vi "Clear Mutation History of lvClass.vi"(8 "error in (no error)":errorcluster, 11 "Path":path=path "D:/OneDrive - NI/_WorkingOn/CSM/Communicable-State-Machine/src/user.lib/_NEVSTOP/Communicable State Machine(CSM)/_Support/Priority Queue/Priority Queue.lvclass") -> (0 "error out":errorcluster, 2 "Mutation History":T1 {"LabVIEW Version" format="%.0x"})   [LabVIEW 2017]
doc: "Clears the mutation history stored in the LabVIEW class at Path and returns the history records that were removed."
uses:
  <vilib>/Utility/EditLVLibs/LVClass/Mutation History.ctl
  <vilib>/Utility/EditLVLibs/LVClass/Mutation Record.ctl
  <vilib>/Utility/EditLVLibs/LibVersion.ctl
  <vilib>/Utility/EditLVLibs/Edit LVLibs.lvlib
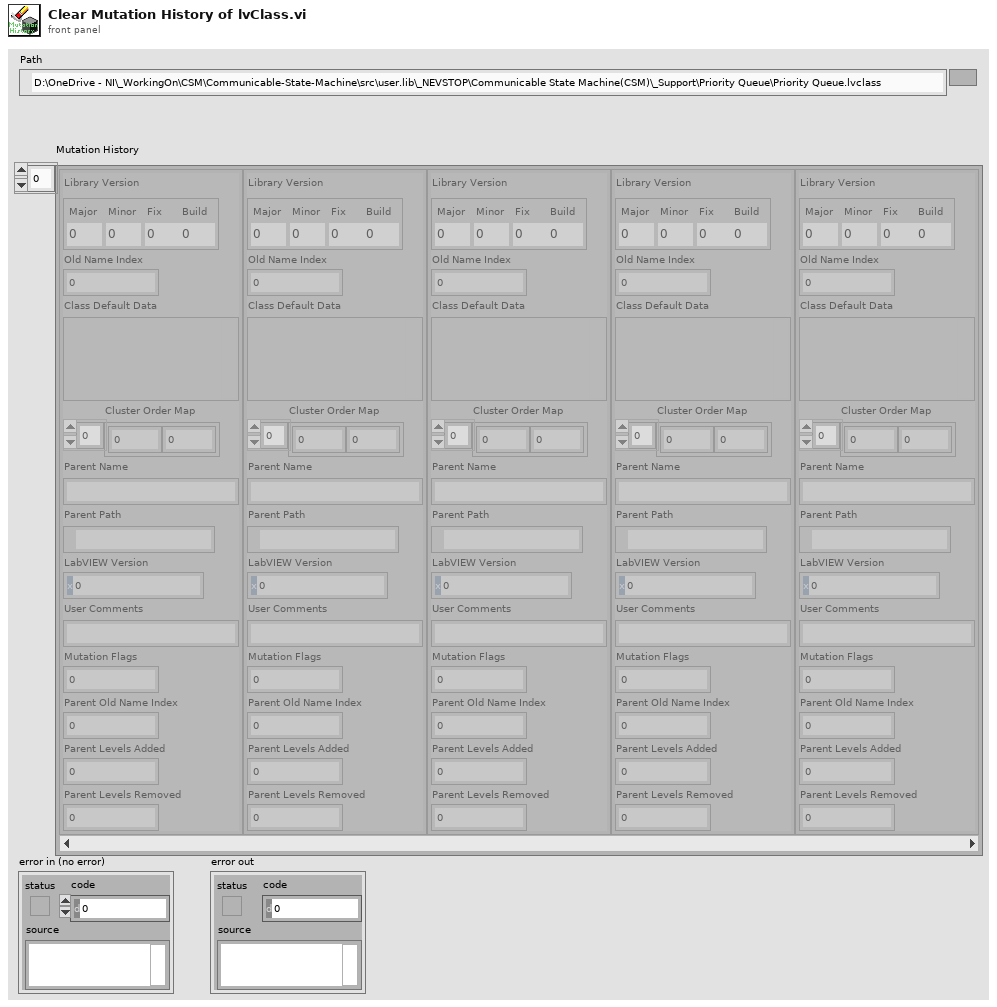
[diagram p1: front panel]
types:
  T1 = typedef "Edit LVLibs.lvlib/Mutation History.ctl" = T2[]
  T2 = typedef "Edit LVLibs.lvlib/Mutation Record.ctl" = cluster{"Library Version":T3, "Old Name Index":u8, "Class Default Data":variant, "Cluster Order Map":u32[], "Parent Name":string, "Parent Path":path, "LabVIEW Version":u32, "User Comments":string, "Mutation Flags":u8, "Parent Old Name Index":u8, "Parent Levels Added":u16, "Parent Levels Removed":u16}
  T3 = typedef "Edit LVLibs.lvlib/LibVersion.ctl" = cluster{"Major":u16, "Minor":u16, "Fix":u16, "Build":u16}
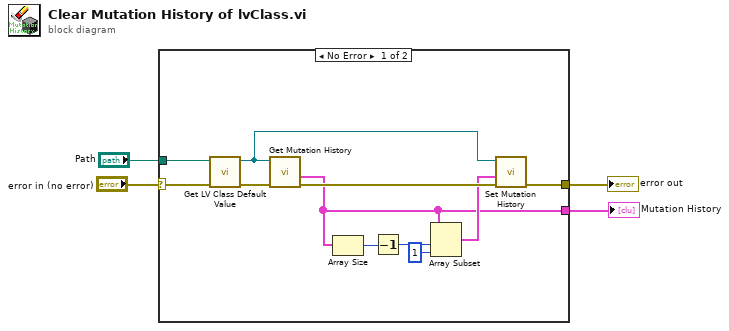
[diagram p0: block diagram]
diagram:
  n1 = case shown="No Error" "error in (no error)" {
    selector: "error in (no error)" -> [w6 w16]
    tunnel: "Path" -> [w14 _]
    tunnel: [w8 _] -> w3
    tunnel: [w5 w16] -> w1
    frame No Error {
      n2 = call <vilib>:"Get LV Class Default Value.vi"("error in (no error)"=w6, "class path"=w14) -> ("error out"=w13:errorcluster, "object"=w11:refnum<class>)  [unwired: 8 in]
      n3 = call <vilib>:"Get Mutation History.vi"("error in"=w13, "Input object"=w11) -> ("error out"=w15:errorcluster, "Mutation History"=w8:T1)  [unwired: 6 in]
      n4 = Array Size(array=w8) -> (size(s)=w10:i32)
      n5 = Decrement(x=w10) -> (x-1=w7:i32)
      n6 = Array Subset(array=w8, index=w7, length=1) -> (w12:T1)
      n7 = call <vilib>:"Set Mutation History.vi"("error in"=w15, "Mutation History"=w12, "Input object"=w11) -> ("error out"=w5:errorcluster)  [unwired: 8 in]
    }
    frame Error {
    }
  }
  "Mutation History" <- w3
  "error out" <- w1
